vi "S7COMM - Parse Response.vi"(7 "Variable Type":T1=enum."BIT", 8 "error in (no error)":errorcluster, 10 "S7 PDU Data":T2 format="0x%02x", 11 "S7":refnum<class "S7NetCom.lvclass">) -> (0 "error out":errorcluster, 1 "Sequence Number":u16, 2 "Data Array":i32[][](array[numeric]), 3 "S7 out":refnum<class "S7NetCom.lvclass">)   [LabVIEW 2014, in "S7NetCom.lvclass"]
doc: "Parses the PLC's response packet (S7 PDU).\n\n#todo: tidy and enhance.\n_____\nCopyright (c) 2019 Hampel Software Engineering (HSE), released under BSD license. More info can be found on https://dokuwiki.hampel-soft.com/code/hse/s7netcom. Original code published by Marc Christenson, Sisu Devices."
uses:
  S7NetCom.lvclass
  Controls/S7NetCom_HexByteArray.ctl
  Controls/S7NetCom_HexByte.ctl
  Controls/S7_Variable_Type.ctl
  S7NetCom.lvclass/S7NetCom.ctl
  S7COMM - Parse Response - Decode Read Item - Split Data Array.vi
  S7COMM - Get Size Factor from Transport Data Type.vi
  S7COMM - Response Item Return Code-error.vi
  S7COMM - Header - Protocol ID--constant.vi
  Accessors/Get Sequence Number.vi
  S7COMM - Evaluate Protocol Header.vi
  S7COMM - Evaluate Message Type.vi
  S7COMM - Evaluate Sequence Number.vi
  S7COMM - Evaluate Response Error Code.vi
  S7COMM - Response Protocol Header Mismatch-error.vi
  S7COMM - Response Message Type Mismatch-error.vi
  S7COMM - Response Sequence Number Mismatch-error.vi
  S7COMM - Response Error Code-error.vi
panel:
  # "More info on https://dokuwiki.hampel-soft.com/code/hse/s7netcom\n\nCopyright (c) 2019, HAMPEL SOFTWARE ENGINEERING (HSE)\nOriginal code developed by Marc Christenson, Sisu Devices\nAll rights reserved.\n\nRedistribution and use in source and binary forms, with or without\nmodification, are permitted provided that the following conditions are met:\n\n1. Redistributions of source code must retain the above copyright\n   notice, this list of conditions and the following disclaimer.\n\n2. Redistributions in binary form must reproduce the above copyright\n   notice, this list of conditions and the following disclaimer in the\n   documentation and/or other materials provided with the distribution.\n\n3. All advertising materials mentioning features or use of this software\n   must display the following acknowledgement:\n   This product includes software developed by HAMPEL SOFTWARE ENGINEERING.\n\n4. Neither the name of HAMPEL SOFTWARE ENGINEERING nor the\n   names of its contributors may be used to endorse or promote products\n   derived from this software without specific prior written permission.\n\nTHIS SOFTWARE IS PROVIDED BY HAMPEL SOFTWARE ENGINEERING ''AS IS'' AND ANY\nEXPRESS OR IMPLIED WARRANTIES, INCLUDING, BUT NOT LIMITED TO, THE IMPLIED\nWARRANTIES OF MERCHANTABILITY AND FITNESS FOR A PARTICULAR PURPOSE ARE\nDISCLAIMED. IN NO EVENT SHALL HAMPEL SOFTWARE ENGINEERING BE LIABLE FOR ANY\nDIRECT, INDIRECT, INCIDENTAL, SPECIAL, EXEMPLARY, OR CONSEQUENTIAL DAMAGES\n(INCLUDING, BUT NOT LIMITED TO, PROCUREMENT OF SUBSTITUTE GOODS OR SERVICES;\nLOSS OF USE, DATA, OR PROFITS; OR BUSINESS INTERRUPTION) HOWEVER CAUSED AND\nON ANY THEORY OF LIABILITY, WHETHER IN CONTRACT, STRICT LIABILITY, OR TORT\n(INCLUDING NEGLIGENCE OR OTHERWISE) ARISING IN ANY WAY OUT OF THE USE OF THIS\nSOFTWARE, EVEN IF ADVISED OF THE POSSIBILITY OF SUCH DAMAGE."
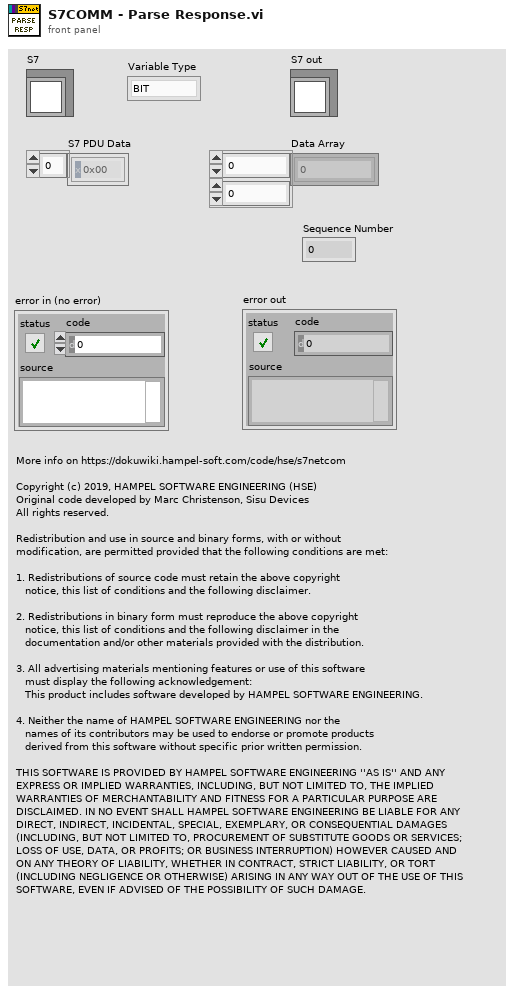
[diagram p1: front panel]
types:
  T1 = typedef "S7NetCom.lvclass/S7_Variable_Type.ctl" = enum8{"---", "BIT", "BYTE", "CHAR", "WORD", "INT", "DWORD", "DINT", "REAL"}
  T2 = typedef "S7NetCom.lvclass/S7NetCom_HexByteArray.ctl" = T3[]
  T3 = typedef "S7NetCom.lvclass/S7NetCom_HexByte.ctl" = u8
  T4 = typedef "S7NetCom.lvclass/S7COMM - Function Codes--ring.ctl" = u8
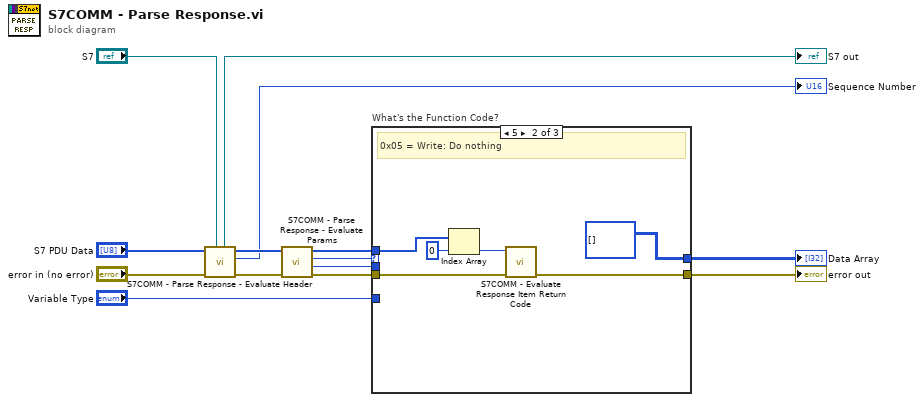
[diagram p0: block diagram]
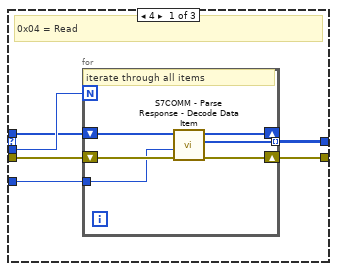
[diagram p2: hidden frame]
diagram:
  n1 = call "S7COMM - Parse Response - Evaluate Header.vi"("S7"="S7", "error in (no error)"="error in (no error)", "S7 PDU Data in"="S7 PDU Data") -> ("error out"=w7:errorcluster, "Sequence Number"=→"Sequence Number":u16, "S7COMM Param and Data"=w8:T2, "S7 out"=→"S7 out":refnum<class "S7NetCom.lvclass">)  [unwired: 5 in]
  n2 = call "S7COMM - Parse Response - Evaluate Params.vi"("error in (no error)"=w7, "S7COMM Params and Data"=w8) -> ("error out"=w3:errorcluster, "Item Count"=w5:T3, "Function Code"=w6:T4, "S7COMM Data"=w4:T2)  [unwired: 6 in]
  n3 = case "What's the Function Code?" shown="5" w6 {
    tunnel: w4 -> [w19 w30 _]
    tunnel: w5 -> [w20 _ _]
    tunnel: [w18 i32[][] [] ("Data Array") _] -> w14
    tunnel: "Variable Type" -> [w17 _ _]
    tunnel: w3 -> [w16 w29 w33]
    tunnel: [w15 w28 w33] -> w2
    frame 4 {
      # "0x04 = Read"
      n4 = for {
        N: w20 -> [_]
        shift-right: [w21] -> _
        shift-left: w19 -> [w25]
        tunnel: [w26] -> w18 mode=indexing
        tunnel: w17 -> [w22]
        shift-right: [w23] -> w15
        shift-left: w16 -> [w24]
        # "iterate through all items"
        n5 = call "S7COMM - Parse Response - Decode Data Item.vi"("error in (no error)"=w24, "Variable Type"=w22, "Response Data IN"=w25) -> ("error out"=w23:errorcluster, "Read Item - Data"=w26:i32[], "Response Data OUT"=w21:T2)  [unwired: 6 in]
      }
    }
    frame 5 {
      # "0x05 = Write: Do nothing"
      n6 = Index Array(array=w30, index=0) -> (element=w27:T3)
      n7 = call "S7COMM - Evaluate Response Item Return Code.vi"("error in (no error)"=w29, "Return Code"=w27) -> ("error out"=w28:errorcluster)  [unwired: 9 in]
    }
    frame Default {
      # "Any other Function Code: Do nothing"
    }
  }
  "Data Array" <- w14
  "error out" <- w2
